vi "test-quintic-spline-03a.vi"() -> (3 "Test Passed":bool)   [LabVIEW 2019]
uses:
  <vilib>/Rock Robotics/WPI/ThirdParty/JAS_Junk/TrajLib/POSEwCURVATURE.ctl
  <vilib>/Rock Robotics/WPI/ThirdParty/JAS_Junk/TrajLib/POSE2D.ctl
  <vilib>/Rock Robotics/WPI/ThirdParty/JAS_Junk/TrajLib/TRANSLATION2D.ctl
  <vilib>/Rock Robotics/WPI/ThirdParty/JAS_Junk/TrajLib/ROTATION2D.ctl
  <vilib>/Rock Robotics/WPI/ThirdParty/JAS_Junk/TrajLib/Rotation_CreateAngle.vi
  <vilib>/Rock Robotics/WPI/ThirdParty/JAS_Junk/TrajLib/Translation_Create.vi
  <vilib>/Rock Robotics/WPI/ThirdParty/JAS_Junk/TrajLib/Util_CalcDist.vi
  <vilib>/Rock Robotics/WPI/ThirdParty/JAS_Junk/TrajLib/Trajectory_Library.lvlib
panel:
  out "XY Graph":cluster{dbl[], dbl[]}(graph)
  out "Numb\nWaypoints":i32
  out "All Interior \nwayPoints\nFound (True)":bool
  out "end rot = 0":dbl
  out "end y = 0":dbl
  out "end x = 0":dbl
  out "start rot = 0":dbl
  out "start y = 0":dbl
  out "start x = 0":dbl
  out "max dtheta < 0.0872":dbl
  out "max dy < 0.00127":dbl
  out "max dx  < 0.127":dbl
  out "Overall Error":errorcluster
  out "Elements":i32
  out "Create Spline Error":errorcluster
  out "SplinePoses\nWCurve":T1[](array[typedef]) {"POSE"."ROTATION"."SIN" format="%13.4f"; "POSE"."ROTATION"."COS" format="%13.4f"; "POSE"."ROTATION"."VALUE" format="%13.4f"; "POSE"."TRANSLATION"."Y" format="%14.3f"; "POSE"."TRANSLATION"."X" format="%14.3f"}
  out "Elapsed Time":dbl
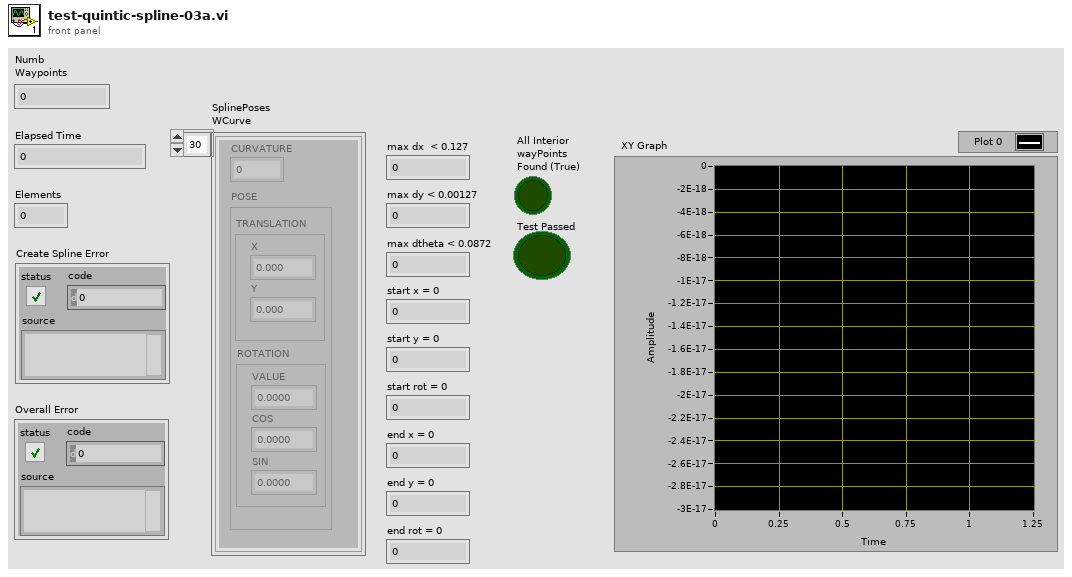
[diagram p1: front panel]
types:
  T1 = typedef "Trajectory_Library.lvlib/POSEwCURVATURE.ctl" = cluster{"CURVATURE":dbl, "POSE":T2}
  T2 = typedef "Trajectory_Library.lvlib/POSE2D.ctl" = cluster{"TRANSLATION":T3, "ROTATION":T4}
  T3 = typedef "Trajectory_Library.lvlib/TRANSLATION2D.ctl" = cluster{"X":dbl, "Y":dbl}
  T4 = typedef "Trajectory_Library.lvlib/ROTATION2D.ctl" = cluster{"VALUE":dbl, "COS":dbl, "SIN":dbl}
  T5 = typedef "Trajectory_Library.lvlib/SPLINE_CTRL_VECTOR.ctl" = cluster{"Xs":dbl[], "Ys":dbl[]}
  T6 = typedef "Trajectory_Library.lvlib/SPLINE.ctl" = cluster{"Degree":i32, "Coefficients":T7}
  T7 = typedef "NI_Matrix.lvlib/RealMatrix.ctl" = dbl[][]
  T8 = typedef "Trajectory_Library.lvlib/TWIST2D.ctl" = cluster{"dX":dbl, "dY":dbl, "dTHETA":dbl}
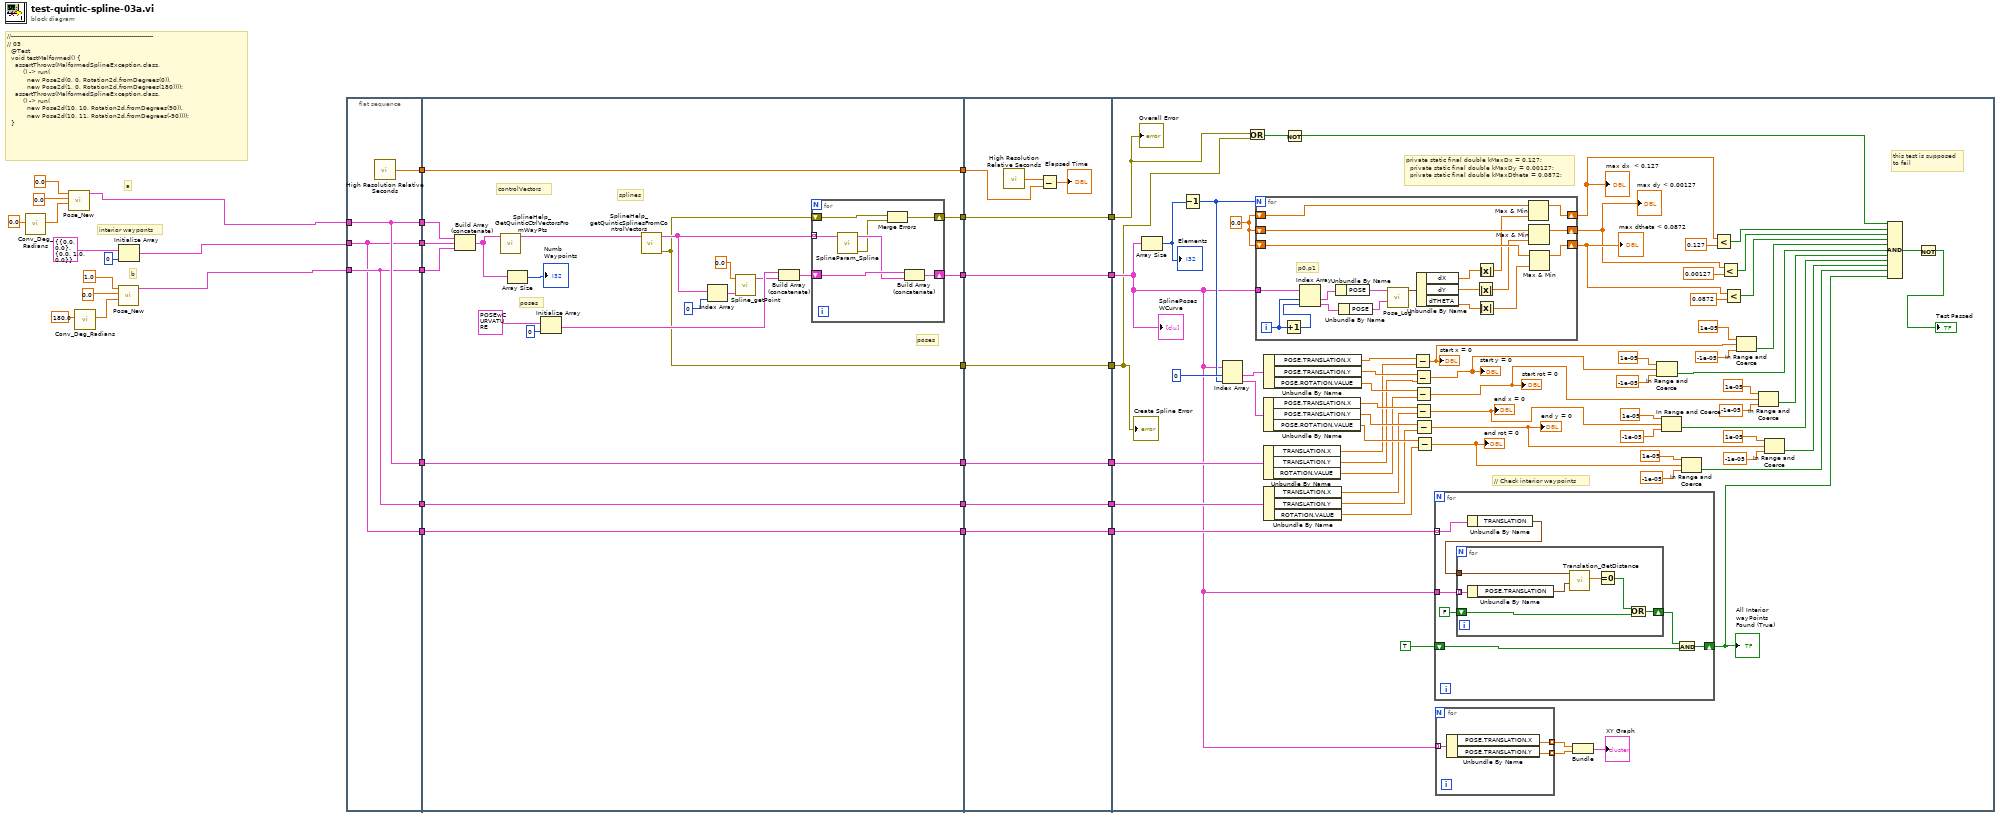
[diagram p0: block diagram]
diagram:
  # "interior wayponts"
  # "b"
  # "a"
  # "//-----------------------------------------------------------------------\n// 03\n  @Test\n  void testMalformed() {\n    assertThrows(MalformedSplineException.class,\n        () -> run(\n          new Pose2d(0, 0, Rotation2d.fromDegrees(0)),\n          new Pose2d(1, 0, Rotation2d.fromDegrees(180))));\n    assertThrows(MalformedSplineException.class,\n        () -> run(\n          new Pose2d(10, 10, Rotation2d.fromDegrees(90)),\n          new Pose2d(10, 11, Rotation2d.fromDegrees(-90))));\n  }"
  n1 = call <vilib>:"Conv_Deg_Radians.vi"("Degress"=0.0) -> ("Radians"=w6:dbl)  [unwired: 10 in]
  n2 = call <vilib>:"Pose_New.vi"("Heading"=w6, "Y"=0.0, "X"=0.0) -> ("out POSe"=w1:T2)  [unwired: 8 in]
  n3 = call <vilib>:"Conv_Deg_Radians.vi"("Degress"=180.0) -> ("Radians"=w9:dbl)  [unwired: 10 in]
  n4 = call <vilib>:"Pose_New.vi"("Heading"=w9, "Y"=0.0, "X"=1.0) -> ("out POSe"=w2:T2)  [unwired: 8 in]
  n5 = Initialize Array(T2 {"TRANSLATION"={"X"=0.0, "Y"=0.0}, "ROTATION"={"VALUE"=0.0, "COS"=1.0, "SIN"=0.0}} ("POSE"), 0 ("dimension size")) -> (w3:T2[])
  n6 = flat-sequence {
    tunnel: w1 -> [w36]
    tunnel: [w36] -> w33
    tunnel: w2 -> [w35]
    tunnel: [w35] -> w32
    tunnel: [w37] -> w31
    tunnel: [w36] -> w23
    tunnel: [w35] -> w20
    tunnel: [w34] -> w15
    tunnel: w3 -> [w34]
    tunnel: [w34] -> w14
    tunnel: w33 -> [w43]
    tunnel: w32 -> [w41]
    tunnel: [w59] -> w30
    tunnel: w31 -> [w59]
    tunnel: [w49] -> w29
    tunnel: [w48] -> w27
    tunnel: [w47] -> w25
    tunnel: w23 -> [w46]
    tunnel: [w46] -> w22
    tunnel: w20 -> [w45]
    tunnel: [w45] -> w19
    tunnel: [w44] -> w16
    tunnel: w15 -> [w44]
    tunnel: w14 -> [w38]
    tunnel: w30 -> [w75]
    tunnel: w29 -> [w74]
    tunnel: [w74] -> w28
    tunnel: w27 -> [w73]
    tunnel: [w73] -> w26
    tunnel: w25 -> [w72]
    tunnel: [w72] -> w24
    tunnel: w22 -> [w69]
    tunnel: [w69] -> w21
    tunnel: w19 -> [w68]
    tunnel: [w68] -> w18
    tunnel: [w67] -> w17
    tunnel: w16 -> [w67]
    tunnel: w28 -> [w117]
    tunnel: w26 -> [w105]
    tunnel: w24 -> [w104]
    tunnel: w21 -> [w139]
    tunnel: w18 -> [w138]
    tunnel: w17 -> [w121]
    frame #0 {
      n7 = call <vilib>:"High Resolution Relative Seconds.vi"() -> ("relative seconds"=w37:dbl)
    }
    frame #1 {
      # "poses"
      # "poses"
      # "splines"
      # "controlVectors"
      n8 = Build Array (concatenate)(w43, w38, w41) -> (w40:T2[])
      n9 = call <vilib>:"SplineHelp_GetQuinticCtrlVectorsFromWayPts.vi"("WayPoints"=w40) -> ("SplineControlVectors"=w42:T5[])  [unwired: 10 in]
      n10 = Array Size(array=w40) -> (size(s)=→"Numb\nWaypoints":i32)
      n11 = Initialize Array(T1 {"CURVATURE"=0.0, "POSE"={"TRANSLATION"={"X"=0.0, "Y"=0.0}, "ROTATION"={"VALUE"=0.0, "COS"=1.0, "SIN"=0.0}}} ("POSEwCURVATURE"), 0 ("dimension size")) -> (w53:T1[])
      n12 = call <vilib>:"SplineHelp_getQuinticSplinesFromControlVectors.vi"("ControlVectors"=w42) -> ("error out"=w48:errorcluster, "splines"=w50:T6[])  [unwired: 9 in]
      n13 = Index Array(array=w50, index=0) -> (element=w55:T6)
      n14 = call <vilib>:"Spline_getPoint.vi"("inputSPLINE"=w55, "Time"=0.0) -> ("POSEwCURVATURE"=w52:T1)  [unwired: 9 in]
      n15 = Build Array (concatenate)(w53, w52) -> (w51:T1[])
      n16 = for {
        shift-right: [w63] -> w49
        shift-left: w51 -> [w65]
        tunnel: w50 -> [w66] mode=indexing
        shift-right: [w61] -> w47
        shift-left: w48 -> [w62]
        n17 = call <vilib>:"SplineParam_Spline.vi"("inputSPLINE"=w66) -> ("error out"=w60:errorcluster, "outputPOSEwCURVATURE"=w64:T1[])  [unwired: 9 in]
        n18 = Merge Errors(w62, w60) -> (w61:errorcluster)
        n19 = Build Array (concatenate)(w65, w64) -> (w63:T1[])
      }
    }
    frame #2 {
      n20 = call <vilib>:"High Resolution Relative Seconds.vi"() -> ("relative seconds"=w70:dbl)
      n21 = Subtract(x=w70, y=w75) -> (x-y=→"Elapsed Time":dbl)
    }
    frame #3 {
      w140 = 0.0
      # "this test is supposed\nto fail"
      # "// Check interior waypoints"
      # "private static final double kMaxDx = 0.127;\n  private static final double kMaxDy = 0.00127;\n  private static final double kMaxDtheta = 0.0872;"
      n22 = Array Size(array=w117) -> (size(s)=w141:i32)
      "Elements" <- w141
      n23 = Decrement(x=w141) -> (x-1=w136:i32)
      n24 = Index Array(array=w117, index #1=0 ("index"), index #2=w136) -> (element #1=w135:T1, element #2=w134:T1)
      n25 = Or(x=w104, y=w105) -> (x .or. y?=w106:bool)
      n26 = for {
        N: w136 -> [_]
        tunnel: w117 -> [w176]
        shift-right: [w167] -> w110
        shift-left: w140 -> [w164]
        shift-right: [w165] -> w112
        shift-left: w140 -> [w162]
        shift-right: [w166] -> w111
        shift-left: w140 -> [w163]
        i -> [w178]
        # "p0,p1"
        n27 = Increment(x=w178) -> (x+1=w177:i32)
        n28 = Index Array(array=w176, index #1=w178, index #2=w177) -> (element #1=w175:T1, element #2=w174:T1)
        n29 = Unbundle By Name(w175) -> ("POSE"=w173:T2)
        n30 = Unbundle By Name(w174) -> ("POSE"=w172:T2)
        n31 = call <vilib>:"Pose_Log.vi"("end POSE"=w172, "in POSE"=w173) -> ("out TWIST"=w171:T8)  [unwired: 9 in]
        n32 = Unbundle By Name(w171) -> ("dX"=w168:dbl, "dY"=w169:dbl, "dTHETA"=w170:dbl)
        n33 = Absolute Value(x=w169) -> (abs(x)=w160:dbl)
        n34 = Absolute Value(x=w168) -> (abs(x)=w161:dbl)
        n35 = Absolute Value(x=w170) -> (abs(x)=w159:dbl)
        n36 = Max & Min(x=w164, y=w161) -> (max(x,y)=w167:dbl)  [unwired: 1 out]
        n37 = Max & Min(x=w163, y=w160) -> (max(x,y)=w166:dbl)  [unwired: 1 out]
        n38 = Max & Min(x=w162, y=w159) -> (max(x,y)=w165:dbl)  [unwired: 1 out]
      }
      "max dx  < 0.127" <- w110
      "max dy < 0.00127" <- w111
      "max dtheta < 0.0872" <- w112
      n39 = Unbundle By Name(w134) -> ("POSE.TRANSLATION.X"=w130:dbl, "POSE.TRANSLATION.Y"=w129:dbl, "POSE.ROTATION.VALUE"=w128:dbl)
      n40 = Unbundle By Name(w139) -> ("TRANSLATION.X"=w127:dbl, "TRANSLATION.Y"=w126:dbl, "ROTATION.VALUE"=w125:dbl)
      n41 = Unbundle By Name(w135) -> ("POSE.TRANSLATION.X"=w133:dbl, "POSE.TRANSLATION.Y"=w132:dbl, "POSE.ROTATION.VALUE"=w131:dbl)
      n42 = Unbundle By Name(w138) -> ("TRANSLATION.X"=w124:dbl, "TRANSLATION.Y"=w123:dbl, "ROTATION.VALUE"=w122:dbl)
      n43 = Not(x=w106) -> (.not. x?=w103:bool)
      n44 = Subtract(x=w133, y=w127) -> (x-y=w99:dbl)
      "start x = 0" <- w99
      n45 = Subtract(x=w132, y=w126) -> (x-y=w78:dbl)
      "start y = 0" <- w78
      n46 = Subtract(x=w131, y=w125) -> (x-y=w82:dbl)
      "start rot = 0" <- w82
      n47 = Subtract(x=w130, y=w124) -> (x-y=w83:dbl)
      "end x = 0" <- w83
      n48 = Subtract(x=w129, y=w123) -> (x-y=w90:dbl)
      "end y = 0" <- w90
      n49 = Subtract(x=w128, y=w122) -> (x-y=w94:dbl)
      "end rot = 0" <- w94
      n50 = for {
        tunnel: w121 -> [w146] mode=indexing
        tunnel: w117 -> [w151]
        shift-right: [w150] -> w102
        shift-left: TRUE -> [w149]
        n51 = Unbundle By Name(w146) -> ("TRANSLATION"=w145:T3)
        n52 = for {
          tunnel: w151 -> [w155] mode=indexing
          shift-right: [w158] -> w147
          shift-left: FALSE -> [w157]
          tunnel: w145 -> [w156]
          n53 = Unbundle By Name(w155) -> ("POSE.TRANSLATION"=w154:T3)
          n54 = call <vilib>:"Translation_GetDistance.vi"("other Translation"=w154, "In Translation"=w156) -> ("Distance"=w153:dbl)  [unwired: 9 in]
          n55 = Equal To 0?(x=w153) -> (x = 0?=w152:bool)
          n56 = Or(x=w152, y=w157) -> (x .or. y?=w158:bool)
        }
        n57 = And(x=w147, y=w149) -> (x .and. y?=w150:bool)
      }
      "All Interior \nwayPoints\nFound (True)" <- w102
      n58 = for {
        tunnel: [w144] -> w119 mode=indexing
        tunnel: [w143] -> w118 mode=indexing
        tunnel: w117 -> [w142] mode=indexing
        n59 = Unbundle By Name(w142) -> ("POSE.TRANSLATION.X"=w144:dbl, "POSE.TRANSLATION.Y"=w143:dbl)
      }
      n60 = Bundle(w119, w118) -> (→"XY Graph":cluster{dbl[], dbl[]})  [unwired: 1 in]
      n61 = In Range and Coerce(upper limit=1e-05, x=w78, lower limit=-1e-05) -> (In Range?=w79:bool)  [unwired: 1 out]
      n62 = In Range and Coerce(upper limit=1e-05, x=w83, lower limit=-1e-05) -> (In Range?=w85:bool)  [unwired: 1 out]
      n63 = In Range and Coerce(upper limit=1e-05, x=w94, lower limit=-1e-05) -> (In Range?=w95:bool)  [unwired: 1 out]
      n64 = Less?(x=w110, y=0.127) -> (x < y?=w109:bool)
      n65 = Less?(x=w111, y=0.00127) -> (x < y?=w108:bool)
      n66 = Less?(x=w112, y=0.0872) -> (x < y?=w107:bool)
      n67 = In Range and Coerce(upper limit=1e-05, x=w99, lower limit=-1e-05) -> (In Range?=w98:bool)  [unwired: 1 out]
      n68 = In Range and Coerce(upper limit=1e-05, x=w82, lower limit=-1e-05) -> (In Range?=w84:bool)  [unwired: 1 out]
      n69 = In Range and Coerce(upper limit=1e-05, x=w90, lower limit=-1e-05) -> (In Range?=w91:bool)  [unwired: 1 out]
      n70 = Compound Arithmetic op=AND(w103, w109, w108, w107, w98, w79, w84, w85, w91, w95, w102) -> (w77:bool)
      n71 = Not(x=w77) -> (.not. x?=→"Test Passed":bool)
      "SplinePoses\nWCurve" <- w117
      "Create Spline Error" <- w105
      "Overall Error" <- w104
    }
  }
